vi "Check_Traverse_move.vi"(0 "Current position":dbl[](array[numeric])=[0.0, 0.0, 0.0] format="%.2f", 1 "Traverse Name":string, 2 "Full Check":bool, 5 "New Position":dbl[](array[numeric])=[0.0, 0.0, 0.0] format="%.2f", 7 "Coordinate rotation (deg)":dbl format="%.2f", 9 "Probe Volume":T2=[{"Max"=15.0, "Min"=-15.0}, {"Max"=250.0, "Min"=0.0}, {"Max"=15.0, "Min"=-15.0}] {"Min" format="%#.1f"; "Max" format="%#.1f"}, 11 "Entire Space":T2=[{"Max"=15001.0, "Min"=12000.0}, {"Max"=1000.0, "Min"=-1000.0}, {"Max"=700.0, "Min"=0.0}] {"Min" format="%#.1f"; "Max" format="%#.1f"}, 12 "Exclude Array":T1[](array[typedef])=[{"Sizes"=[{"Max"=15000.0, "Min"=0.0}, {"Max"=1000.0, "Min"=-1000.0}, {"Max"=300.0, "Min"=0.0}], "Name"="Roughness Elements", "Exclude Type"=enum."Allow only vertical moves"}, {"Sizes"=[{"Max"=17000.0, "Min"=16000.0}, {"Max"=200.0, "Min"=-200.0}, {"Max"=-50.0, "Min"=-250.0}], "Name"="B204", "Exclude Type"=enum."Exclude completely"}] {"Sizes"."Min" format="%#.1f"; "Sizes"."Max" format="%#.1f"}) -> (6 "Position At Crash":dbl[](array[numeric]) format="%.2f", 10 "Steps":dbl[][](array[numeric]) format="%.2f", 15 "Error Comments":string)   [LabVIEW 2010]
uses:
  Box_size.ctl
  Exclude_cluster.ctl
  Exclusion_type.ctl
panel:
  # "X                Y                   Z"
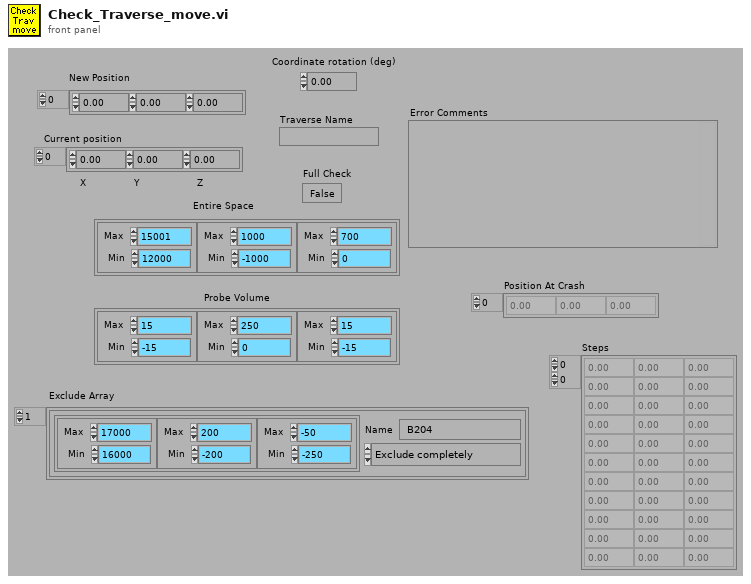
[diagram p1: front panel]
types:
  T1 = typedef "Exclude_cluster.ctl" = cluster{"Sizes":T2, "Name":string, "Exclude Type":T3}
  T2 = typedef "Box_size.ctl" = cluster{"Max":dbl, "Min":dbl}[]
  T3 = typedef "Exclusion_type.ctl" = enum16{"Exclude completely", "Allow only vertical moves"}
  T4 = enum16{"To Traverse Coordinates", "To User Coordinates"}
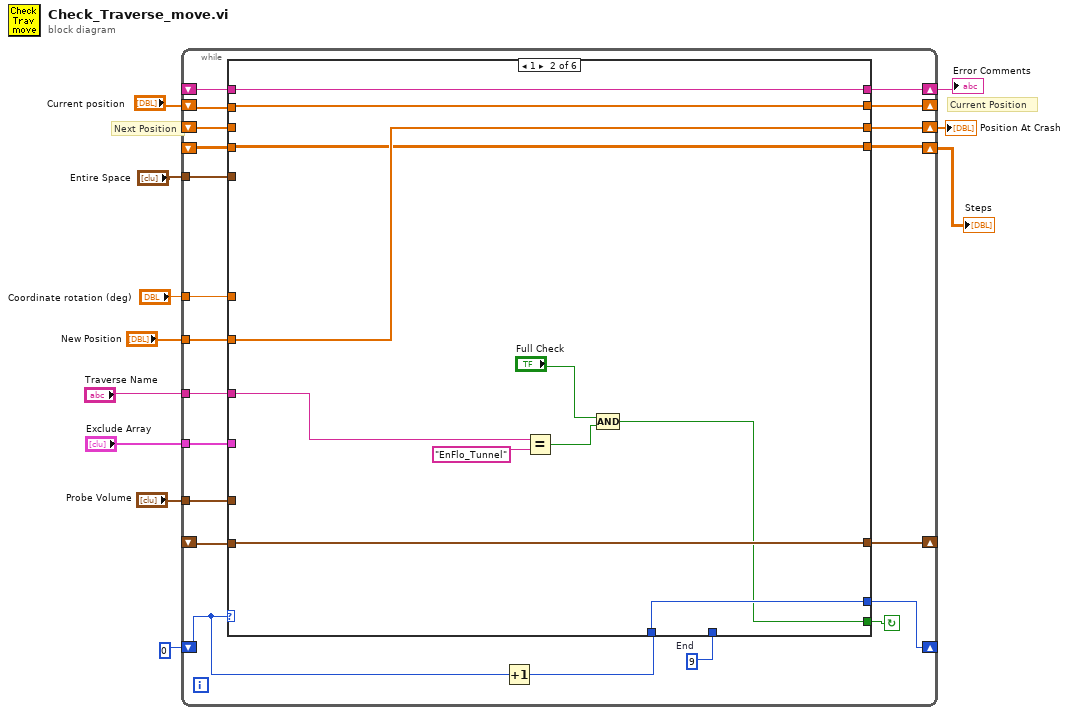
[diagram p0: block diagram]
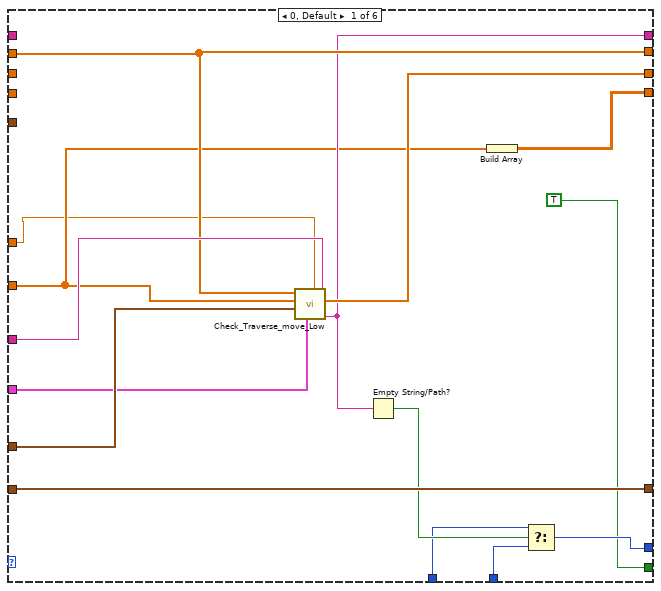
[diagram p2: hidden frame]
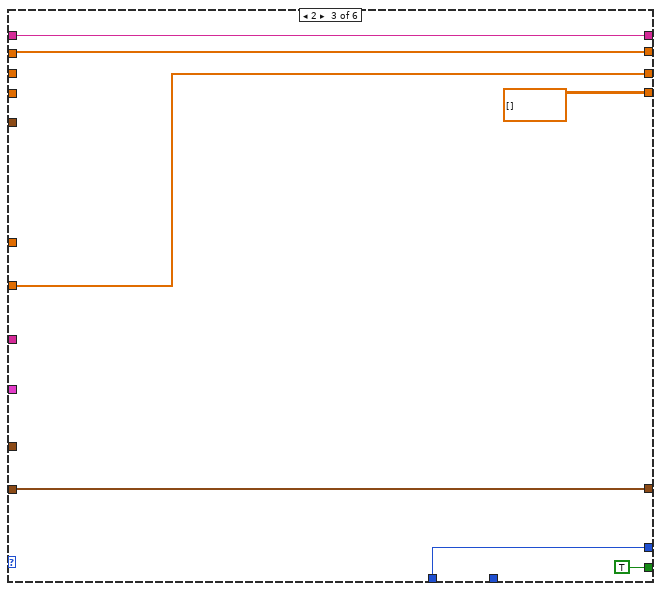
[diagram p3: hidden frame]
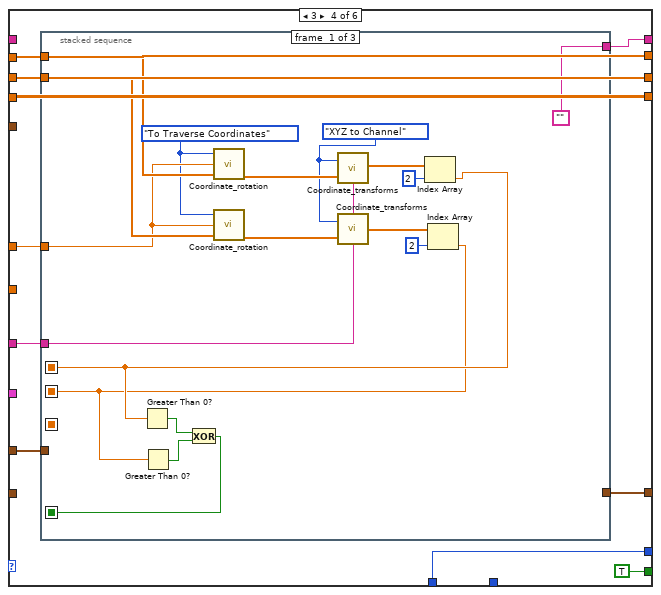
[diagram p4: hidden frame]
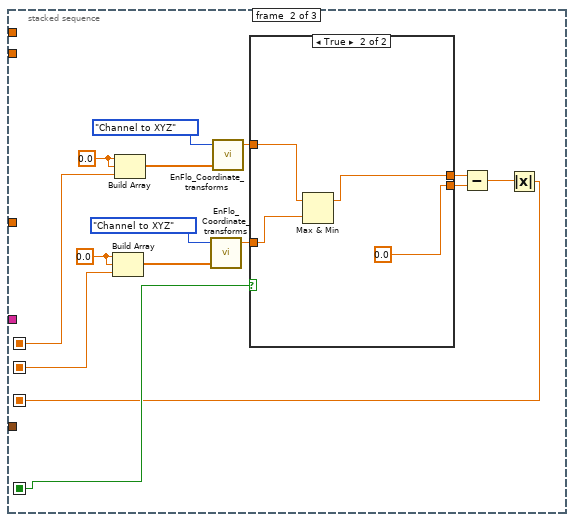
[diagram p5: hidden frame]
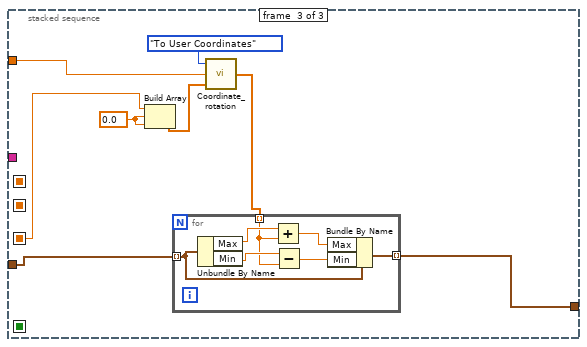
[diagram p7: hidden frame]
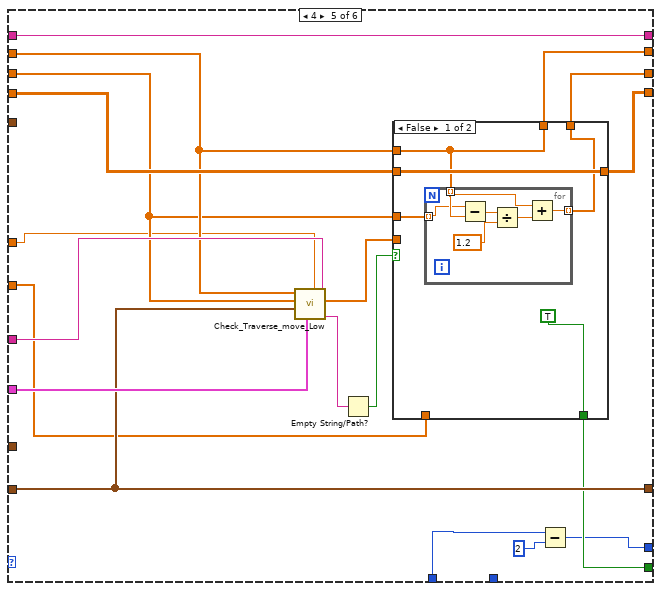
[diagram p8: hidden frame]
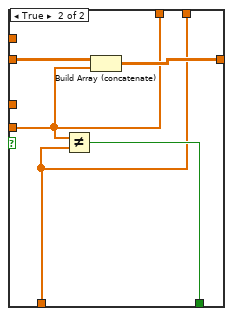
[diagram p9: hidden frame]
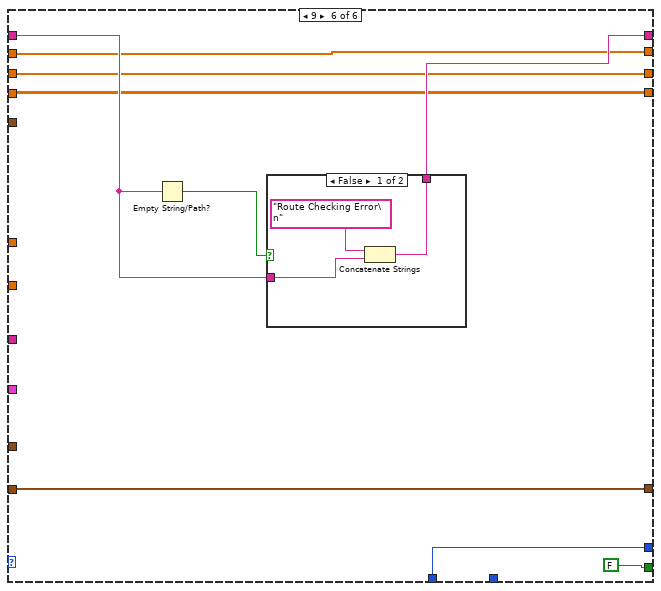
[diagram p10: hidden frame]
diagram:
  # "Current Position"
  # "Next Position"
  n1 = while {
    shift-left: _ -> [w13]
    shift-right: [w12] -> w1
    tunnel: "Probe Volume" -> [w15]
    shift-left: _ -> [w17]
    shift-right: [w16] -> _
    tunnel: "Coordinate rotation (deg)" -> [w18]
    tunnel: "New Position" -> [w19]
    shift-left: _ -> [w21]
    shift-right: [w22] -> w6
    shift-left: 0 -> [w25]
    shift-right: [w24] -> _
    tunnel: "Traverse Name" -> [w26]
    tunnel: "Entire Space" -> [w27]
    tunnel: "Exclude Array" -> [w28]
    shift-left: _ -> [w20]
    shift-right: [w30] -> w4
    shift-left: "Current position" -> [w32]
    shift-right: [w31] -> _
    stop <- w29 continue-if-true
    w14 = 9  # End
    n2 = Increment(x=w25) -> (x+1=w23:i32)
    n3 = case shown="1" w25 {
      tunnel: w32 -> [w42 w57 w64 w72 w132 w167]
      tunnel: [w42 w57 w64 w72 w137 w167] -> w31
      tunnel: [w45 w50 w61 w71 w136 w166] -> w30
      tunnel: [TRUE ("Box Inside") w52 TRUE ("Box Inside") TRUE ("Box Inside") w139 FALSE ("Box Inside")] -> w29
      tunnel: w17 -> [w44 w56 w63 _ w146 w168]
      tunnel: w28 -> [w46 _ _ _ w148 _]
      tunnel: w27 -> [_ _ _ _ _ _]
      tunnel: w26 -> [w43 w53 _ w69 w147 _]
      tunnel: [w37 w55 w62 w67 w134 w170] -> w24
      tunnel: w23 -> [w39 w55 w62 w67 w133 w170]
      tunnel: [w41 w58 w65 w75 w144 w171] -> w22
      tunnel: w21 -> [_ w58 w65 _ w144 w172]
      tunnel: w20 -> [_ _ _ w71 w131 w166]
      tunnel: w19 -> [w36 w50 w61 _ w140 _]
      tunnel: w18 -> [w34 _ _ w70 w130 _]
      tunnel: [w44 w56 w63 w73 w146 w168] -> w16
      tunnel: w15 -> [w47 _ _ w68 _ _]
      tunnel: w14 -> [w38 _ _ _ _ _]
      tunnel: w13 -> [_ w49 _ w66 w143 w165]
      tunnel: [w35 w49 dbl[][] [] w66 w142 w165] -> w12
      frame 0, Default {
        n4 = call "Check_Traverse_move_Low.vi"("Traverse Name"=w43, "Rotation (deg)"=w34, "Exclude Array"=w46, "Probe Volume"=w47, "New Position"=w36, "Current position"=w42) -> ("Error Comments"=w41:string, "Position At Crash"=w45:dbl[])  [unwired: 2 out]
        n5 = Empty String/Path?(string/path=w41) -> (empty?=w40:bool)
        n6 = Build Array(w36) -> (w35:dbl[][])
        n7 = Select(t=w39, s=w40, f=w38) -> (s? t:f=w37:i32)
      }
      frame 1 {
        n8 = Equal?(x=w53, y="EnFlo_Tunnel") -> (x = y?=w48:bool)
        n9 = Compound Arithmetic op=AND("Full Check", w48) -> (w52:bool)
      }
      frame 2 {
      }
      frame 3 {
        n10 = stacked-sequence {
          seq-local: [w78 _ _] -> [_ w108 _]
          seq-local: [w77 _ _] -> [_ w107 _]
          seq-local: [w76 _ _] -> [_ w98 _]
          seq-local: [_ w94 _] -> [_ _ w117]
          tunnel: ["" _ _] -> w75
          tunnel: [_ _ w121] -> w73
          tunnel: w72 -> [w91 _ _]
          tunnel: w71 -> [w89 _ _]
          tunnel: w70 -> [w88 _ w115]
          tunnel: w69 -> [w87 _ _]
          tunnel: w68 -> [_ _ w122]
          frame #0 {
            w85 = enum16{"XYZ to Channel", "Channel to XYZ"}."XYZ to Channel" ("Mode")
            w86 = T4."To Traverse Coordinates" ("Mode")
            n11 = call "Coordinate_rotation.vi"("Input Position"=w91, "Coordinate rotation (deg)"=w88, "Mode"=w86) -> ("Output Position"=w92:dbl[])
            n12 = call "Coordinate_rotation.vi"("Input Position"=w89, "Coordinate rotation (deg)"=w88, "Mode"=w86) -> ("Output Position"=w90:dbl[])
            n13 = call "Coordinate_transforms.vi"("Traverse Name"=w87, "Input"=w92, "Mode"=w85) -> ("Output"=w84:dbl[])
            n14 = call "Coordinate_transforms.vi"("Traverse Name"=w87, "Input"=w90, "Mode"=w85) -> ("Output"=w81:dbl[])
            n15 = Index Array(array=w84, index=2) -> (element=w78:dbl)
            n16 = Greater Than 0?(x=w78) -> (x > 0?=w80:bool)
            n17 = Index Array(array=w81, index=2) -> (element=w77:dbl)
            n18 = Greater Than 0?(x=w77) -> (x > 0?=w79:bool)
            n19 = Exclusive Or(1:w79, 2:w80) -> (0:w76:bool)
          }
          frame #1 {
            w101 = 0.0 ("element")
            w106 = 0.0 ("element")
            n20 = Build Array(w101, w101, w107) -> (w103:dbl[])
            n21 = Build Array(w106, w106, w108) -> (w104:dbl[])
            n22 = call "EnFlo_Coordinate_transforms.vi"("Input"=w103, "Mode"=enum16{"XYZ to Channel", "Channel to XYZ"}."Channel to XYZ") -> ("X theta"=w99:dbl)  [unwired: 3 out]
            n23 = call "EnFlo_Coordinate_transforms.vi"("Input"=w104, "Mode"=enum16{"XYZ to Channel", "Channel to XYZ"}."Channel to XYZ") -> ("X theta"=w100:dbl)  [unwired: 3 out]
            n24 = case shown="True" w98 {
              tunnel: w100 -> [w110 w113]
              tunnel: w99 -> [w109 w114]
              tunnel: [w109 0.0 ("element")] -> w97
              tunnel: [w110 w112] -> w96
              frame False {
              }
              frame True {
                n25 = Max & Min(x=w113, y=w114) -> (max(x,y)=w112:dbl)  [unwired: 1 out]
              }
            }
            n26 = Subtract(x=w96, y=w97) -> (x-y=w95:dbl)
            n27 = Absolute Value(x=w95) -> (abs(x)=w94:dbl)
          }
          frame #2 {
            w119 = 0.0 ("Input Element")
            n28 = Build Array(w117, w119, w119) -> (w118:dbl[])
            n29 = call "Coordinate_rotation.vi"("Input Position"=w118, "Coordinate rotation (deg)"=w115, "Mode"=T4."To User Coordinates") -> ("Output Position"=w116:dbl[])
            n30 = for {
              tunnel: w122 -> [w129] mode=indexing
              tunnel: w116 -> [w124] mode=indexing
              tunnel: [w123] -> w121 mode=indexing
              n31 = Unbundle By Name(w129) -> ("Max"=w128:dbl, "Min"=w127:dbl)
              n32 = Add(x=w128, y=w124) -> (x+y=w126:dbl)
              n33 = Subtract(x=w127, y=w124) -> (x-y=w125:dbl)
              n34 = Bundle By Name(cluster=w129, "Max"=w126, "Min"=w125) -> (w123:cluster{"Max":dbl, "Min":dbl})
            }
          }
        }
      }
      frame 4 {
        n35 = call "Check_Traverse_move_Low.vi"("Traverse Name"=w147, "Rotation (deg)"=w130, "Exclude Array"=w148, "Probe Volume"=w146, "New Position"=w131, "Current position"=w132) -> ("Error Comments"=w145:string, "Position At Crash"=w138:dbl[])  [unwired: 2 out]
        n36 = Empty String/Path?(string/path=w145) -> (empty?=w141:bool)
        n37 = case shown="False" w141 {
          tunnel: w143 -> [w153 w164]
          tunnel: w138 -> [_ w161]
          tunnel: [w153 w163] -> w142
          tunnel: w140 -> [_ w160]
          tunnel: [TRUE w162] -> w139
          tunnel: [w151 w161] -> w137
          tunnel: [w149 w160] -> w136
          tunnel: w132 -> [w151 _]
          tunnel: w131 -> [w150 _]
          frame False {
            n38 = for {
              tunnel: w151 -> [w155] mode=indexing
              tunnel: w150 -> [w154] mode=indexing
              tunnel: [w156] -> w149 mode=indexing
              n39 = Subtract(x=w154, y=w155) -> (x-y=w159:dbl)
              n40 = Divide(x=w159, y=1.2) -> (x/y=w157:dbl)
              n41 = Add(x=w155, y=w157) -> (x+y=w156:dbl)
            }
          }
          frame True {
            n42 = Not Equal?(x=w161, y=w160) -> (x != y?=w162:bool)
            n43 = Build Array (concatenate)(w164, w161) -> (w163:dbl[][])
          }
        }
        n44 = Subtract(x=w133, y=2) -> (x-y=w134:i32)
      }
      frame 9 {
        n45 = Empty String/Path?(string/path=w172) -> (empty?=w173:bool)
        n46 = case shown="False" w173 {
          tunnel: [w174 w177] -> w171
          tunnel: w172 -> [w176 w177]
          frame False {
            n47 = Concatenate Strings("Route Checking Error\n" ("String to match"), w176) -> (w174:string)
          }
          frame True {
          }
        }
      }
    }
  }
  "Error Comments" <- w6
  "Position At Crash" <- w4
  "Steps" <- w1
